vi "DEMO(读取CPU序列号).vi"() -> ()   [LabVIEW 2012]
uses:
  ManagementClass/ManagementClass.lvclass
panel:
  out "propertyValue":string="512"
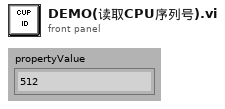
[diagram p1: front panel]
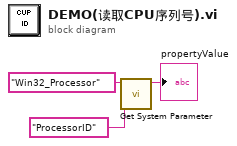
[diagram p0: block diagram]
diagram:
  n1 = call "Get System Parameter.vi"("propertyName"="ProcessorID", "path"="Win32_Processor") -> ("propertyValue"=→"propertyValue":string)  [unwired: 8 in, 1 out]
